vi "not_even_an_event_structure.vi"() -> ()   [LabVIEW 2023]
panel:
  in  "Boolean 25":bool
  in  "stop":bool
  in  "check":bool
  in  "Enum":enum16{"Wait", "Close", "Check"}(ring)
  out "Array":bool[](array[boolean])
  in  "operation":enum16{"AND", "OR", "XOR"}(ring)
  out "Boolean 24":bool
  out "Boolean 23":bool
  out "Boolean 22":bool
  out "Boolean 21":bool
  out "Boolean 20":bool
  out "Boolean 19":bool
  out "Boolean 18":bool
  out "Boolean 17":bool
  in  "Boolean 16":bool
  in  "Boolean 15":bool
  in  "Boolean 14":bool
  in  "Boolean 13":bool
  in  "Boolean 12":bool
  in  "Boolean 11":bool
  in  "Boolean 10":bool
  in  "Boolean 9":bool
  in  "Boolean 8":bool
  in  "Boolean 7":bool
  in  "Boolean 6":bool
  in  "Boolean 5":bool
  in  "Boolean 4":bool
  in  "Boolean 3":bool
  in  "Boolean 2":bool
  in  "Boolean":bool
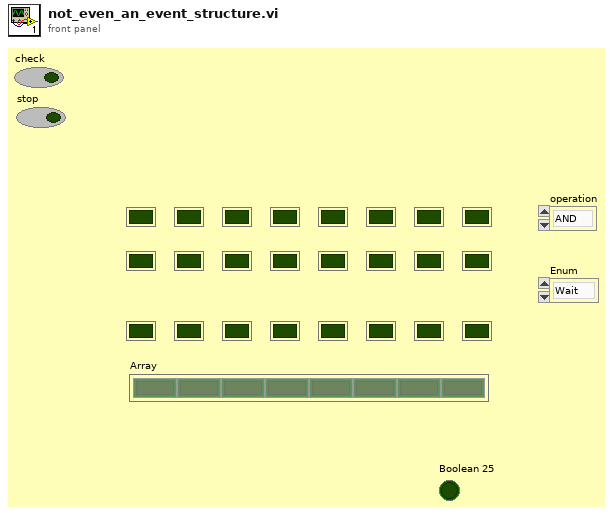
[diagram p1: front panel]
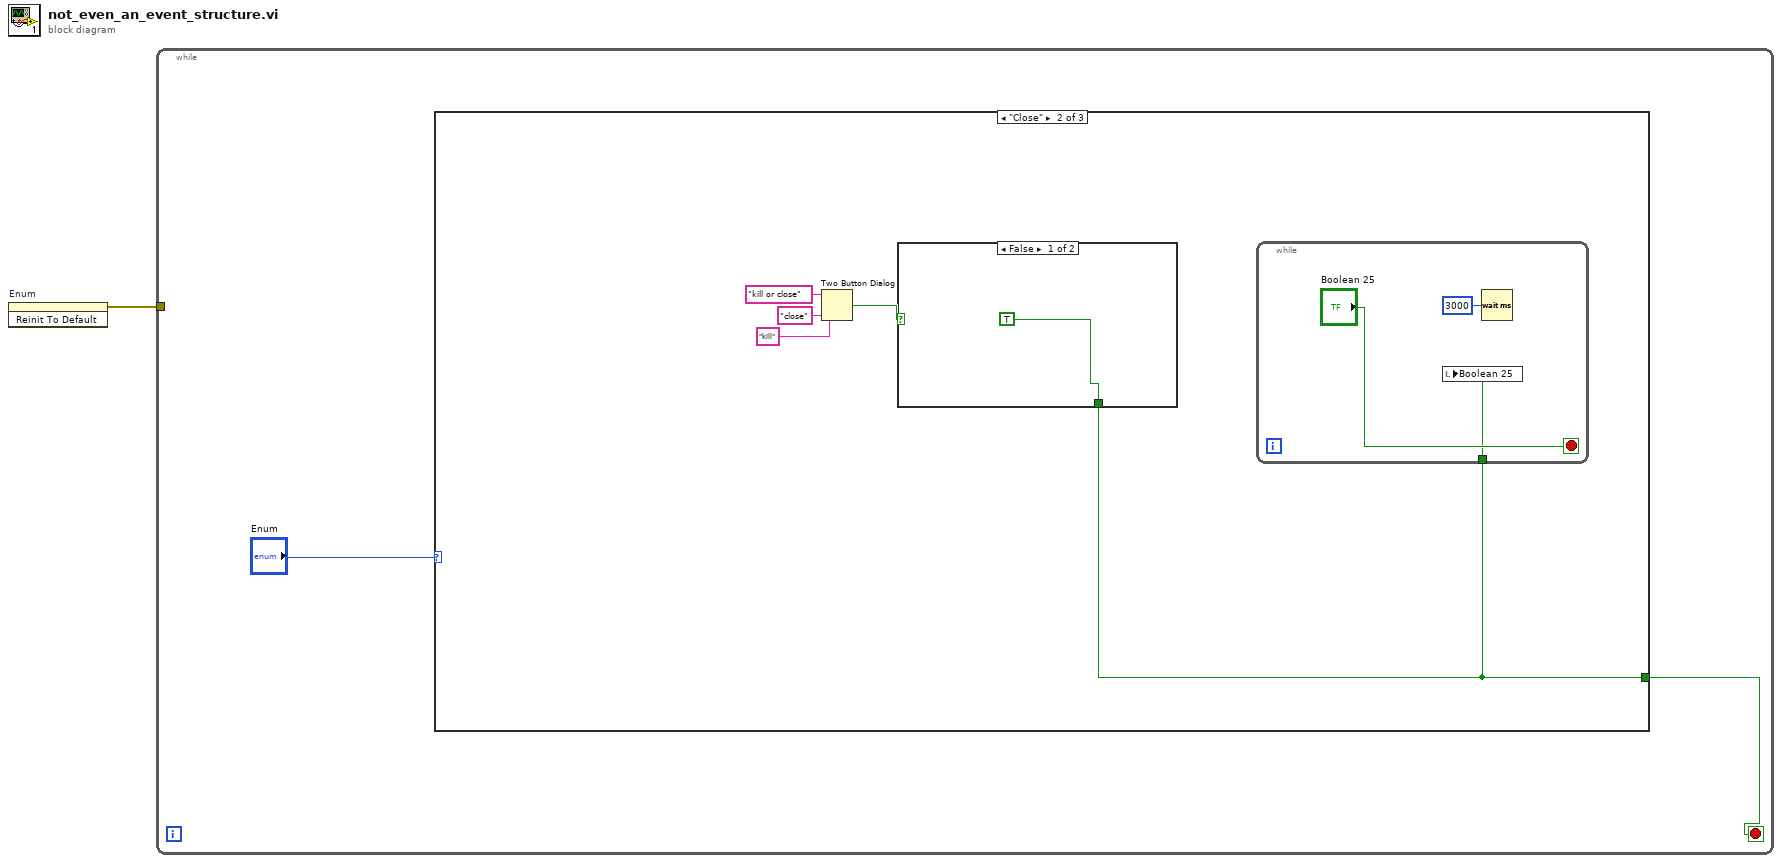
[diagram p0: block diagram]
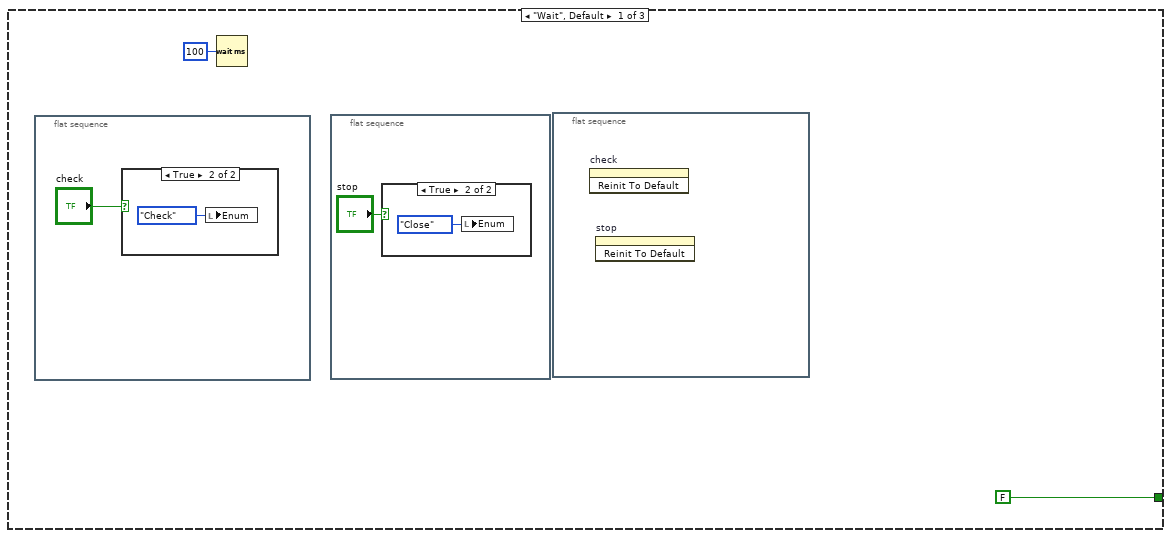
[diagram p2: hidden frame]
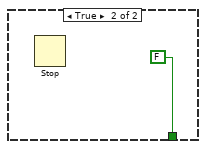
[diagram p5: hidden frame]
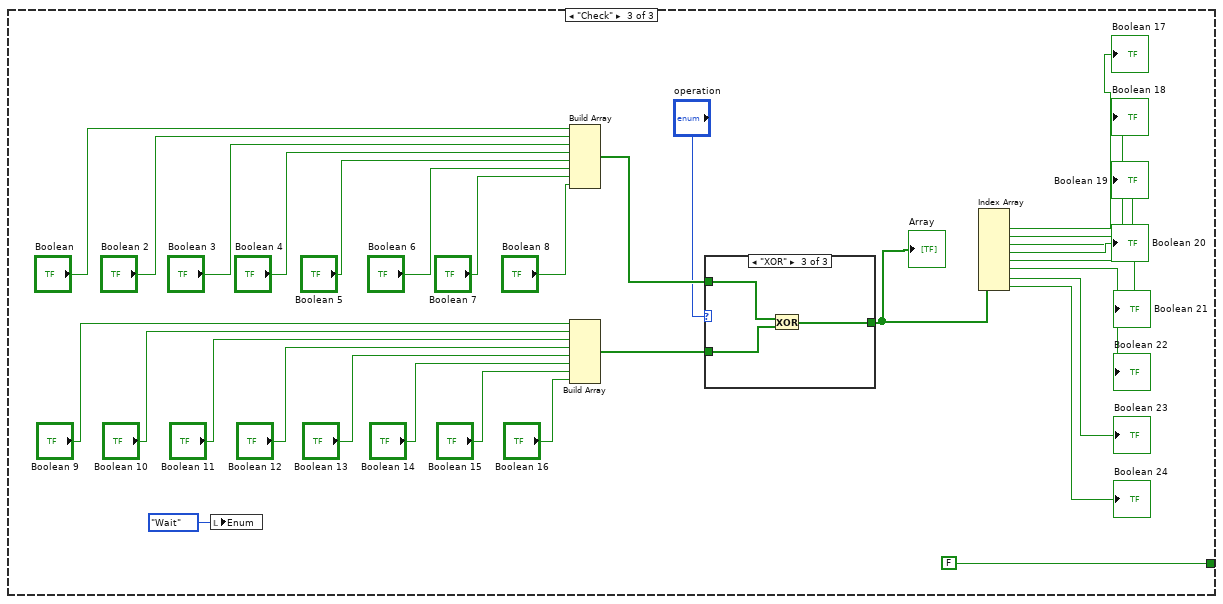
[diagram p6: hidden frame]
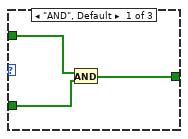
[diagram p7: hidden frame]
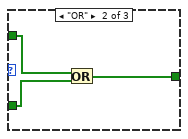
[diagram p8: hidden frame]
diagram:
  n1 = invoke on="Enum" class="Enum (strict)" method="Reinit To Default"() -> (error out=w1:errorcluster)  [unwired: 3 in, 2 out]
  n2 = while {
    tunnel: w1 -> [_]
    stop <- w3 stop-if-true
    n3 = case shown="\"Close\"" "Enum" {
      tunnel: [FALSE w10 FALSE] -> w3
      frame "Wait", Default {
        n4 = flat-sequence {
          frame #0 {
            n5 = case shown="True" "check" {
              frame False {
              }
              frame True {
                n6 = local write "Enum"(enum16{"Wait", "Close", "Check"}."Check" ("Enum")) -> ()
              }
            }
          }
        }
        n7 = Wait (ms)(milliseconds to wait=u32 100) -> ()  [unwired: 1 out]
        n8 = flat-sequence {
          frame #0 {
            n9 = case shown="True" "stop" {
              frame False {
              }
              frame True {
                n10 = local write "Enum"(enum16{"Wait", "Close", "Check"}."Close" ("Enum")) -> ()
              }
            }
          }
        }
        n11 = flat-sequence {
          frame #0 {
            n12 = invoke on="check" class="Bool (strict)" method="Reinit To Default"() -> ()  [unwired: 3 in, 3 out]
            n13 = invoke on="stop" class="Bool (strict)" method="Reinit To Default"() -> ()  [unwired: 3 in, 3 out]
          }
        }
      }
      frame "Close" {
        n14 = Two Button Dialog(message="kill or close", 1:"close" ("F button name (\"Cancel\")"), 2:"kill" ("T button name (\"OK\")")) -> (T button?=w11:bool)
        n15 = case shown="False" w11 {
          tunnel: [TRUE FALSE] -> w10
          frame False {
          }
          frame True {
            n16 = Stop() -> ()  [unwired: 1 in]
          }
        }
        n17 = while {
          tunnel: w10 -> [w16]
          stop <- "Boolean 25" stop-if-true
          n18 = local write "Boolean 25"(w16) -> ()
          n19 = Wait (ms)(milliseconds to wait=u32 3000) -> ()  [unwired: 1 out]
        }
      }
      frame "Check" {
        n20 = local write "Enum"(enum16{"Wait", "Close", "Check"}."Wait" ("Enum")) -> ()
        n21 = Build Array("Boolean", "Boolean 2", "Boolean 3", "Boolean 4", "Boolean 5", "Boolean 6", "Boolean 7", "Boolean 8") -> (w32:bool[])
        n22 = Build Array("Boolean 9", "Boolean 10", "Boolean 11", "Boolean 12", "Boolean 13", "Boolean 14", "Boolean 15", "Boolean 16") -> (w33:bool[])
        n23 = case shown="\"XOR\"" "operation" {
          tunnel: w33 -> [w51 w55 w57]
          tunnel: w32 -> [w52 w54 w58]
          tunnel: [w50 w53 w56] -> w31
          frame "AND", Default {
            n24 = And(x=w52, y=w51) -> (x .and. y?=w50:bool[])
          }
          frame "OR" {
            n25 = Or(x=w54, y=w55) -> (x .or. y?=w53:bool[])
          }
          frame "XOR" {
            n26 = Exclusive Or(1:w57, 2:w58) -> (0:w56:bool[])
          }
        }
        "Array" <- w31
        n27 = Index Array(array=w31) -> (element #1=→"Boolean 17":bool, element #2=→"Boolean 18":bool, element #3=→"Boolean 19":bool, element #4=→"Boolean 20":bool, element #5=→"Boolean 21":bool, element #6=→"Boolean 22":bool, element #7=→"Boolean 23":bool, element #8=→"Boolean 24":bool)  [unwired: 8 in]
      }
    }
  }
